vi "Divide using Coregen(SGL).vi"(8 "Input Valid":bool, 9 "Line Status In":T2, 10 "Divisor":i32, 11 "Dividend":i32[](array[numeric])=[0, 0, 0, 0]) -> (0 "Output Valid":bool, 1 "Line Status Out":T2, 3 "All Channel Data":T3, 4 "Output":cluster{"Output":i16[], "Output Valid":bool})   [LabVIEW 2014]
doc: "<b> Latency = 40 Ticks </b>"
uses:
  <vilib>/rvi/FXPMathLib/basic elements/FxpDiscreteDelay/XNode/nifxpmath_DiscreteDelay.xnode
  Adapter Module Specific/Multi-Channel Analog Input Data.ctl
  Acquisition Engine/Acquisition Status.ctl
panel:
  # "Copyright 2014 Vidrio Technologies\nScanImage 5 software is licensed under the Apache License, Version 2.0 (the \"License\"); you may not use any files contained\nwithin the ScanImage 5 release except in compliance with the License. You may obtain a copy of the License at\n http://www.apache.org/licenses/LICENSE-2.0\nUnless required by applicable law or agreed to in writing, software distributed under the License is distributed on an\n\"AS IS\" BASIS, WITHOUT WARRANTIES OR CONDITIONS OF ANY KIND, either express or implied. See the License for the\n specific language governing permissions and limitations under the License."
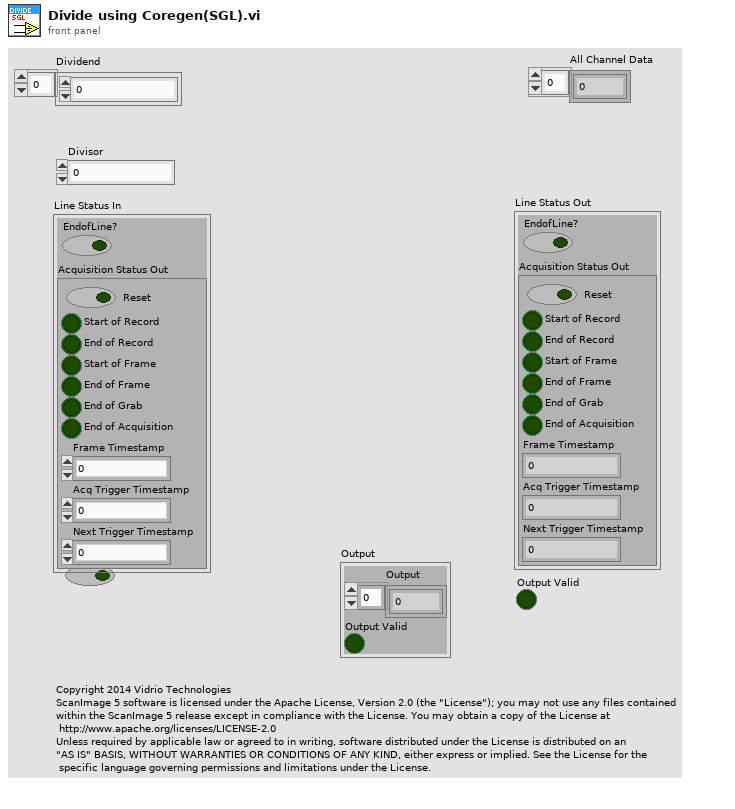
[diagram p1: front panel]
types:
  T1 = typedef "Acquisition Status.ctl" = cluster{"Reset":bool, "Start of Record":bool, "End of Record":bool, "Start of Frame":bool, "End of Frame":bool, "End of Grab":bool, "End of Acquisition":bool, "Frame Timestamp":u64, "Acq Trigger Timestamp":u64, "Next Trigger Timestamp":u64}
  T2 = cluster{"EndofLine?":bool, "Acquisition Status Out":T1}
  T3 = typedef "Multi-Channel Analog Input Data.ctl" = i16[]
  T4 = cluster{"EndofLine?":bool, "Acquisition Status Out":cluster{"Reset":bool, "Start of Record":bool, "End of Record":bool, "Start of Frame":bool, "End of Frame":bool, "End of Grab":bool, "End of Acquisition":bool, "Frame Timestamp":u64, "Acq Trigger Timestamp":u64, "Next Trigger Timestamp":u64}}
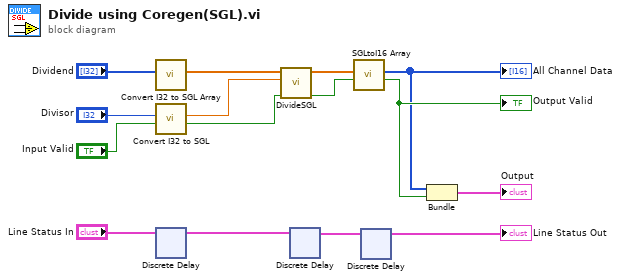
[diagram p0: block diagram]
diagram:
  n1 = call "Convert I32 to SGL Array.vi"("Input (I32)"="Dividend") -> ("Output (SGL)"=w7:sgl[])  [unwired: 9 in, 1 out]
  n2 = call "Convert I32 to SGL.vi"("Input Valid"="Input Valid", "Input (I32)"="Divisor") -> ("Output Valid"=w13:bool, "Output (SGL)"=w12:sgl)  [unwired: 8 in]
  n3 = xnode "Discrete Delay"("D"="Line Status In") -> ("Q"=w10:T4)
  n4 = call "DivideSGL.vi"("Input Valid"=w13, "b"=w12, "a"=w7) -> ("Output Valid"=w1:bool, "a/b"=w6:sgl[])  [unwired: 7 in]
  n5 = xnode "Discrete Delay"("D"=w10) -> ("Q"=w9:T4)
  n6 = call "SGLtoI16 Array.vi"("Input Valid"=w1, "Input"=w6) -> ("Output Valid"=w5:bool, "Output"=w4:i16[])  [unwired: 8 in]
  "Output Valid" <- w5
  "All Channel Data" <- w4
  n7 = xnode "Discrete Delay"("D"=w9) -> ("Q"=→"Line Status Out":T4)
  n8 = Bundle("Output"=w4, "Output Valid"=w5) -> (→"Output":cluster{"Output":i16[], "Output Valid":bool})  [unwired: 1 in]
